vi "prepare.vi"(8 "error in (no error)":errorcluster, 11 "GenericSweep in":refnum<class "GenericSweep.lvclass">) -> (0 "error out":errorcluster, 3 "GenericSweep out":refnum<class "GenericSweep.lvclass">)   [LabVIEW 2010, in "GenericSweep.lvclass"]
uses:
  GenericSweep.lvclass
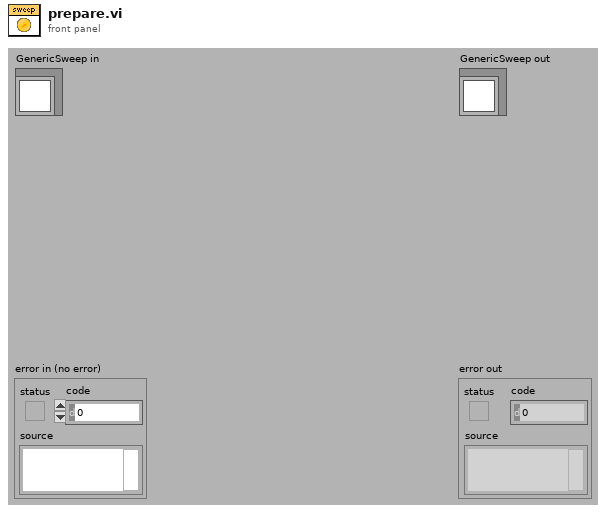
[diagram p1: front panel]
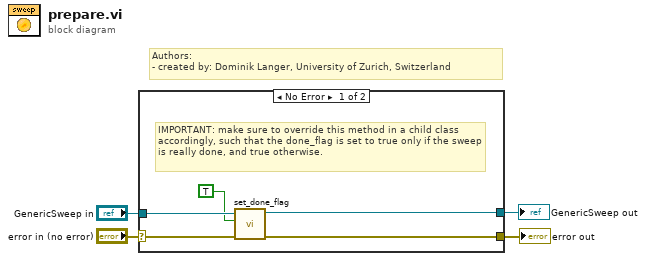
[diagram p0: block diagram]
diagram:
  # "Authors: \n- created by: Dominik Langer, University of Zurich, Switzerland"
  n1 = case shown="No Error" "error in (no error)" {
    selector: "error in (no error)" -> [w6 w11]
    tunnel: [w5 w11] -> w3
    tunnel: [w8 w10] -> w1
    tunnel: "GenericSweep in" -> [w9 w10]
    frame No Error {
      # "IMPORTANT: make sure to override this method in a child class accordingly, such that the done_flag is set to true only if the sweep is really done, and true otherwise."
      n2 = call-dynamic "set_done_flag.vi"("error in (no error)"=w6, "done?"=TRUE, "GenericSweep in"=w9) -> ("error out"=w5:errorcluster, "GenericSweep out"=w8:refnum<class "GenericSweep.lvclass">)  [unwired: 7 in]
    }
    frame Error {
    }
  }
  "error out" <- w3
  "GenericSweep out" <- w1
